vi "svx_Check Mismatch.vi"(7 "reset in":bool, 8 "error in (no error)":errorcluster, 11 "channel property in":T1[](array[typedef]) {"probe angle [deg]" max=360; "direction" items=["CCW", "CW"]}) -> (0 "error out":errorcluster, 2 "pair index":cluster{"index 1":i32, "index 2":i32}[](array[cluster]), 3 "channel property out":T1[](array[typedef]) {"probe angle [deg]" max=360; "direction" items=["CCW", "CW"]}, 5 "reset out":bool)   [LabVIEW 2017]
uses:
  <vilib>/addons/Sound and Vibration/Order Analysis/Data Presentation/SubVIs/OAT MCM Channel Property.ctl
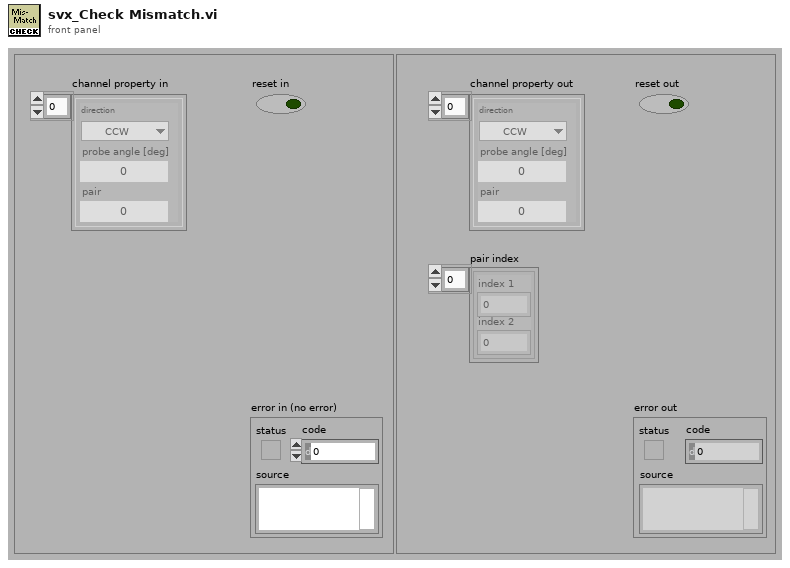
[diagram p1: front panel]
types:
  T1 = typedef "OAT MCM Channel Property.ctl" = cluster{"direction":u16, "probe angle [deg]":u16, "pair":u16}
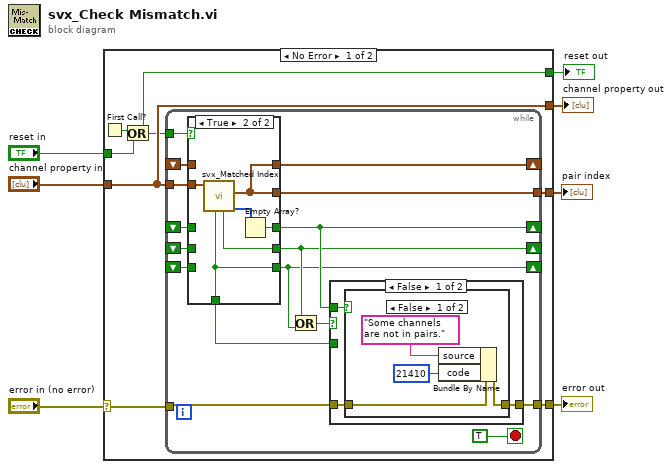
[diagram p0: block diagram]
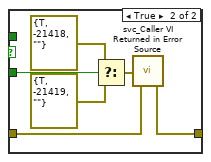
[diagram p3: hidden frame]
diagram:
  n1 = case shown="No Error" "error in (no error)" {
    selector: "error in (no error)" -> [w12 w55]
    tunnel: [w11 w55] -> w6
    tunnel: "reset in" -> [w13 _]
    tunnel: "channel property in" -> [w9 _]
    tunnel: [w10 _] -> w3
    tunnel: [w9 _] -> w2
    tunnel: [w8 _] -> w1
    frame No Error {
      n2 = First Call?() -> (First Call?: T/F=w14:bool)
      n3 = Or(x=w14, y=w13) -> (x .or. y?=w8:bool)
      n4 = while {
        tunnel: w12 -> [w21]
        tunnel: [w20] -> w11
        tunnel: w8 -> [w30]
        tunnel: w9 -> [w29]
        shift-right: [w26] -> _
        shift-left: _ -> [w25]
        tunnel: [w27] -> w10
        shift-right: [w22] -> _
        shift-left: _ -> [w24]
        shift-right: [w17] -> _
        shift-left: _ -> [w23]
        shift-right: [w16] -> _
        shift-left: _ -> [w18]
        stop <- TRUE stop-if-true
        n5 = case shown="True" w30 {
          tunnel: w29 -> [_ w54]
          tunnel: [w48 w53] -> w27
          tunnel: [w48 w53] -> w26
          tunnel: w25 -> [w48 _]
          tunnel: [w47 w51] -> w22
          tunnel: w24 -> [w47 _]
          tunnel: w23 -> [w46 _]
          tunnel: [w45 w49] -> w19
          tunnel: [w46 w50] -> w17
          tunnel: [w45 w49] -> w16
          tunnel: w18 -> [w45 _]
          frame False {
          }
          frame True {
            n6 = call <vilib>:"svx_Matched Index.vi"("channel property"=w54) -> ("single index"=w52:i32[], "pair index"=w53:cluster{"index 1":i32, "index 2":i32}[], "direction error"=w50:bool, "pair error"=w49:bool)  [unwired: 5 in, 2 out]
            n7 = Empty Array?(array=w52) -> (empty?=w51:bool)
          }
        }
        n8 = Or(x=w17, y=w16) -> (x .or. y?=w15:bool)
        n9 = case shown="False" w15 {
          tunnel: w21 -> [w32 w44]
          tunnel: [w31 w43] -> w20
          tunnel: w22 -> [w33 _]
          tunnel: w19 -> [_ w42]
          frame False {
            n10 = case shown="False" w33 {
              tunnel: w32 -> [w37 w38]
              tunnel: [w36 w38] -> w31
              frame False {
                n11 = Bundle By Name(cluster=w37, "source"="Some channels are not in pairs.", "code"=21410) -> (w36:errorcluster)
              }
              frame True {
              }
            }
          }
          frame True {
            n12 = Select(t=errorcluster {"status"=TRUE, "code"=-21418, "source"=""} ("error in (no error)"), s=w42, f=errorcluster {"status"=TRUE, "code"=-21419, "source"=""} ("error in (no error)")) -> (s? t:f=w39:errorcluster)
            n13 = call <vilib>:"svc_Caller VI Returned in Error Source.vi"("warning input to caller"=w44, "error in (no error)"=w39) -> ("error out"=w43:errorcluster)  [unwired: 3 in]
          }
        }
      }
    }
    frame Error {
    }
  }
  "error out" <- w6
  "pair index" <- w3
  "channel property out" <- w2
  "reset out" <- w1
